vi "EmergencyStop.vi"(0 "object in":refnum<class "TowerLight.lvclass">, 2 "Emergency":bool, 5 "error in (no error)":errorcluster) -> (14 "object out":refnum<class "TowerLight.lvclass">, 19 "error out":errorcluster)   [LabVIEW 2014, in "TowerLight.lvclass"]
uses:
  TowerLight.lvclass
  TowerLight.lvclass/TowerLight.ctl
  TrafficLight.ctl
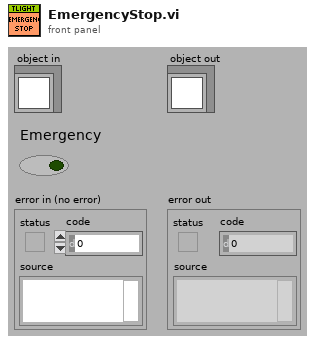
[diagram p1: front panel]
types:
  T1 = typedef "TowerLight.lvclass/TrafficLight.ctl" = cluster{"Red":bool, "Yellow":bool, "Green":bool}
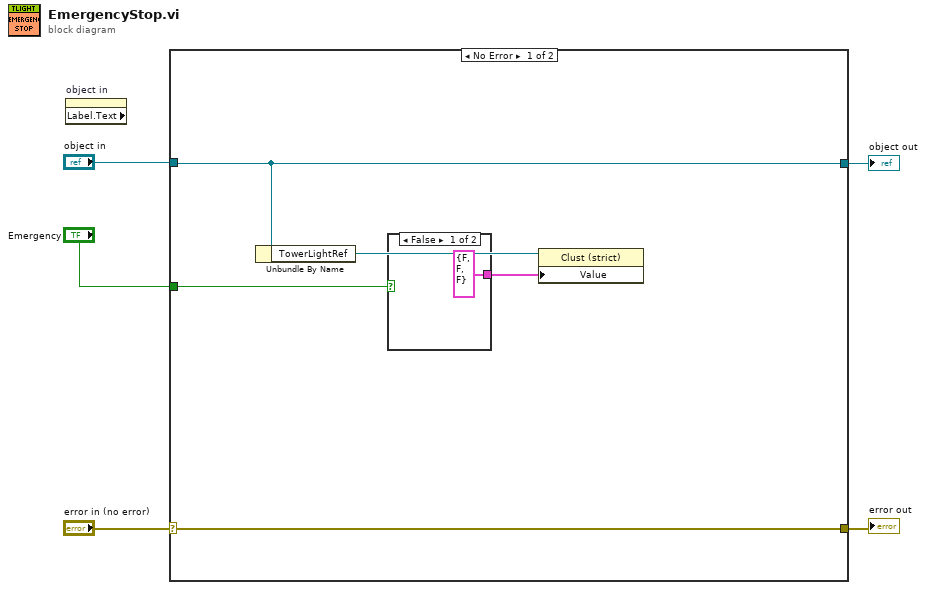
[diagram p0: block diagram]
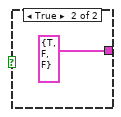
[diagram p2: hidden frame]
diagram:
  n1 = property on="object in" class="LVClassControl (strict)" props=["Label", "Text"]() -> ()  [unwired: 2 in, 3 out]
  n2 = case shown="No Error" "error in (no error)" {
    selector: "error in (no error)" -> [w10 w14]
    tunnel: [w10 w14] -> w4
    tunnel: [w9 w13] -> w2
    tunnel: "object in" -> [w9 w13]
    tunnel: "Emergency" -> [w6 _]
    frame No Error {
      n3 = Unbundle By Name(w9) -> ("TowerLightRef"=w8:refnum<vi>)
      n4 = case shown="False" w6 {
        tunnel: [T1 {"Red"=FALSE, "Yellow"=FALSE, "Green"=FALSE} ("Value") T1 {"Red"=TRUE, "Yellow"=FALSE, "Green"=FALSE} ("Value")] -> w7
        frame False {
        }
        frame True {
        }
      }
      n5 = property class="Clust (strict)"(reference=w8, "Value"=w7) -> ()  [unwired: 1 in, 2 out]
    }
    frame Error {
    }
  }
  "error out" <- w4
  "object out" <- w2
